vi "手动3界面.vi"(8 "错误输入（无错误）":errorcluster, 10 "界面切换队列":refnum<queue>, 11 "VISA资源名称输入":refnum<visa-resource-name>) -> (0 "错误输出":errorcluster, 3 "VISA资源名称输出":refnum<visa-resource-name>)   [LabVIEW 2018]
panel:
  out "DT470+上限+主料盘第三个":dbl
  out "DT469+下限+主料盘第三个":dbl
  out "DT468+上限+主料盘第二个":dbl
  out "DT467+下限+主料盘第二个":dbl
  out "R3":bool
  out "毫秒计时值":u32
  in  "枚举":T1(ring)
  in  "选项卡控件":enum32{"选项卡 1", "选项卡 2"}(tab)
  out "写R2E+读Y1C+2号吸嘴真空":bool
  out "写R2C+读Y1B+1号吸嘴真空":bool
  out "写R66+读R67+Z2下降取料":bool
  out "写R62+读R63+Z1下降取料":bool
  out "写R1F+读R5F+R2轴旋转定位":bool
  out "写R1C+读R5C+R1轴旋转定位":bool
  out "写R6C+读R6D+Z轴校正位取料":bool
  out "写R64+读R65+XYZ2到2号飞达位":bool
  out "写R60+读R61+XYZ1到飞达位":bool
  out "写R6A+读R6B+Z轴校正位放料":bool
  out "写R3F+读R4F+Z2下降编带":bool
  out "写R3D+读R4D+Z1下降编带":bool
  out "写R37+读R47+Z2下降取料":bool
  out "写R168+读R168+切换+快速":bool
  out "写R35+读R45+Z1下降取料":bool
  out "写R68+读R69+XY到校正位":bool
  out "写R3E+读R4E+XYZ2到2号编带位":bool
  out "写R3C+读R4C+XYZ1到1号编带位":bool
  out "写R36+读R46+XYZ2到指定点":bool
  out "写DT676+主料盘第3个":dbl
  out "写DT670+主料盘第2个":dbl
  out "写DDT600+主料盘已取个数":dbl
  out "手动2界面":bool
  out "DDT90356":dbl
  out "DDT90348":dbl
  out "自动界面":bool
  out "手动界面":bool
  out "参数界面":bool
  out "IO界面":bool
  out "产品界面":bool
  out "字符串":string
  out "DDT90352":dbl
  out "DDT90360":dbl
  out "DT1184":T2(ring)
  out "写R0+读R1+手动启动":bool
  out "写R4+读R4+手动停止":bool
  out "写R8+读R9+机器复位":bool
  out "写R80+读R80+报警清除":bool
  out "手动4界面":bool
  out "通讯周期":dbl
  in  "DT62+枚举":enum16{"90度", "180度", "270度"}(ring)
  in  "DT63+枚举":enum16{"90度", "180度", "270度"}(ring)
  out "写R76+读R76+主料盘修改":bool
  out "写R81+读R81+切换+快速":bool
  out "写R34+读R44+XYZ1到指定点":bool
  # "X"
  # "Z1"
  # "Z2"
  # "Y"
  # "备\n料\n盘\n状\n态"
  # "已取"
  # "个"
  # "第"
  # "行"
  # "第"
  # "个"
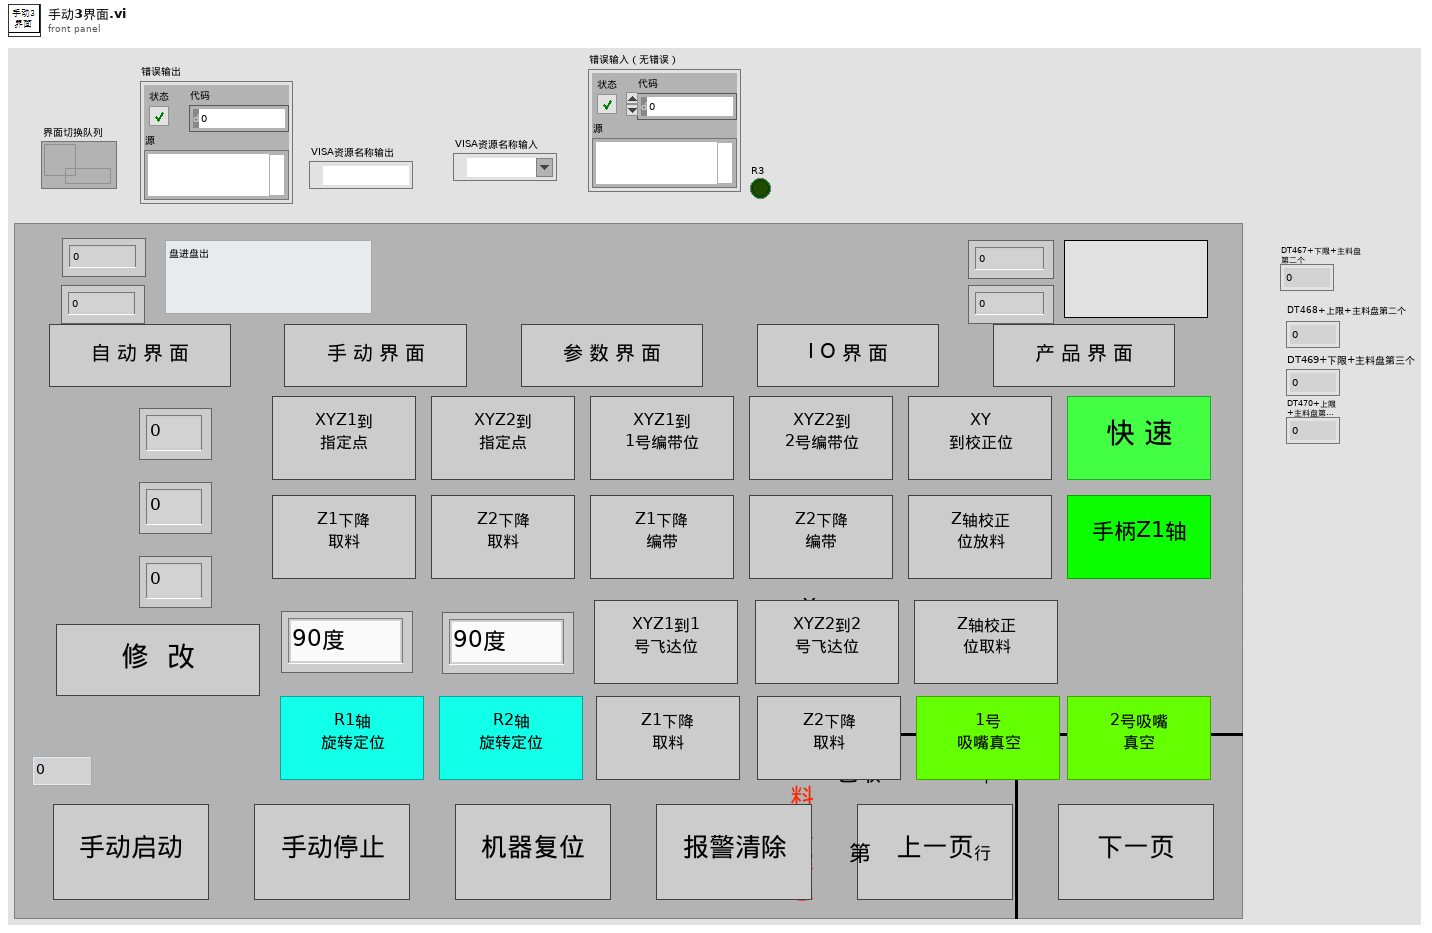
[diagram p1: front panel]
types:
  T1 = enum16{"读初始化", "读DT467+10", "读R4C+8", "读R44+8", "读R61+8", "读R75+8", "读R168+8", "读Y1B+8", "读R80+8", "读R69+8", "读R5C+8", "读R9+8", "读R1+8", "读DT670+10", "读DDT600+5", "读DT1184", "读DT62+10", "读DDT90356", "读DDT90348", ""}
  T2 = enum16{"盘进盘出", "卷进卷出", "盘进卷出", "管进盘出", "管进卷出", "卷进盘出", ""}
  T3 = typedef "数据簇.ctl" = cluster{"字符串":string, "数值":i32, "布尔":bool}
  T4 = enum8{"Enabled", "Disabled", "Disabled and Grayed Out"}
  T5 = typedef "lveventtype.ctl" = enum32{"Null", "Timeout", "Annotation Menu Selection", "Annotation Menu Selection?", "App Instance Close", "App Instance Close?", "Autoscale Range Change", "Bookmark Info Change", "Cell Edit", "Cell Edit?", "Cursor Grab", "Cursor Grab?", "Cursor Menu Selection", "Cursor Menu Selection?", "Cursor Move", "Cursor Release", "Data Change", "Direction Change", "Display State Change", "Drag Ended", "Drag Enter", "Drag Leave", "Drag Over", "Drag Source Update", "Drag Starting", "Drag Starting?", "Drop", "Exec State Change", "Key Down", "Key Down?", "Key Repeat", "Key Repeat?", "Key Up", "Listbox Double Click", "Menu Activation?", "Menu Selection (App)", "Menu Selection? (App)", "Menu Selection (User)", "Mouse Down", "Mouse Down?", "Mouse Enter", "Mouse Leave", "Mouse Move", "Mouse Up", "Mouse Wheel", "NI Security User Change (App)", "Pane Size", "Panel Close", "Panel Close?", "Panel Resize", "Plot Attribute Change", "Scale Range Change", "Shortcut Menu Activation?", "Shortcut Menu Selection (App)", "Shortcut Menu Selection? (App)", "Shortcut Menu Selection (User)", "Tree Double Click", "Tree Drag", "Tree Drag?", "Tree Drop", "Tree Drop?", "Tree Item Close", "Tree Item Close?", "Tree Item Open", "Tree Item Open?", "User Event", "Value Change"}
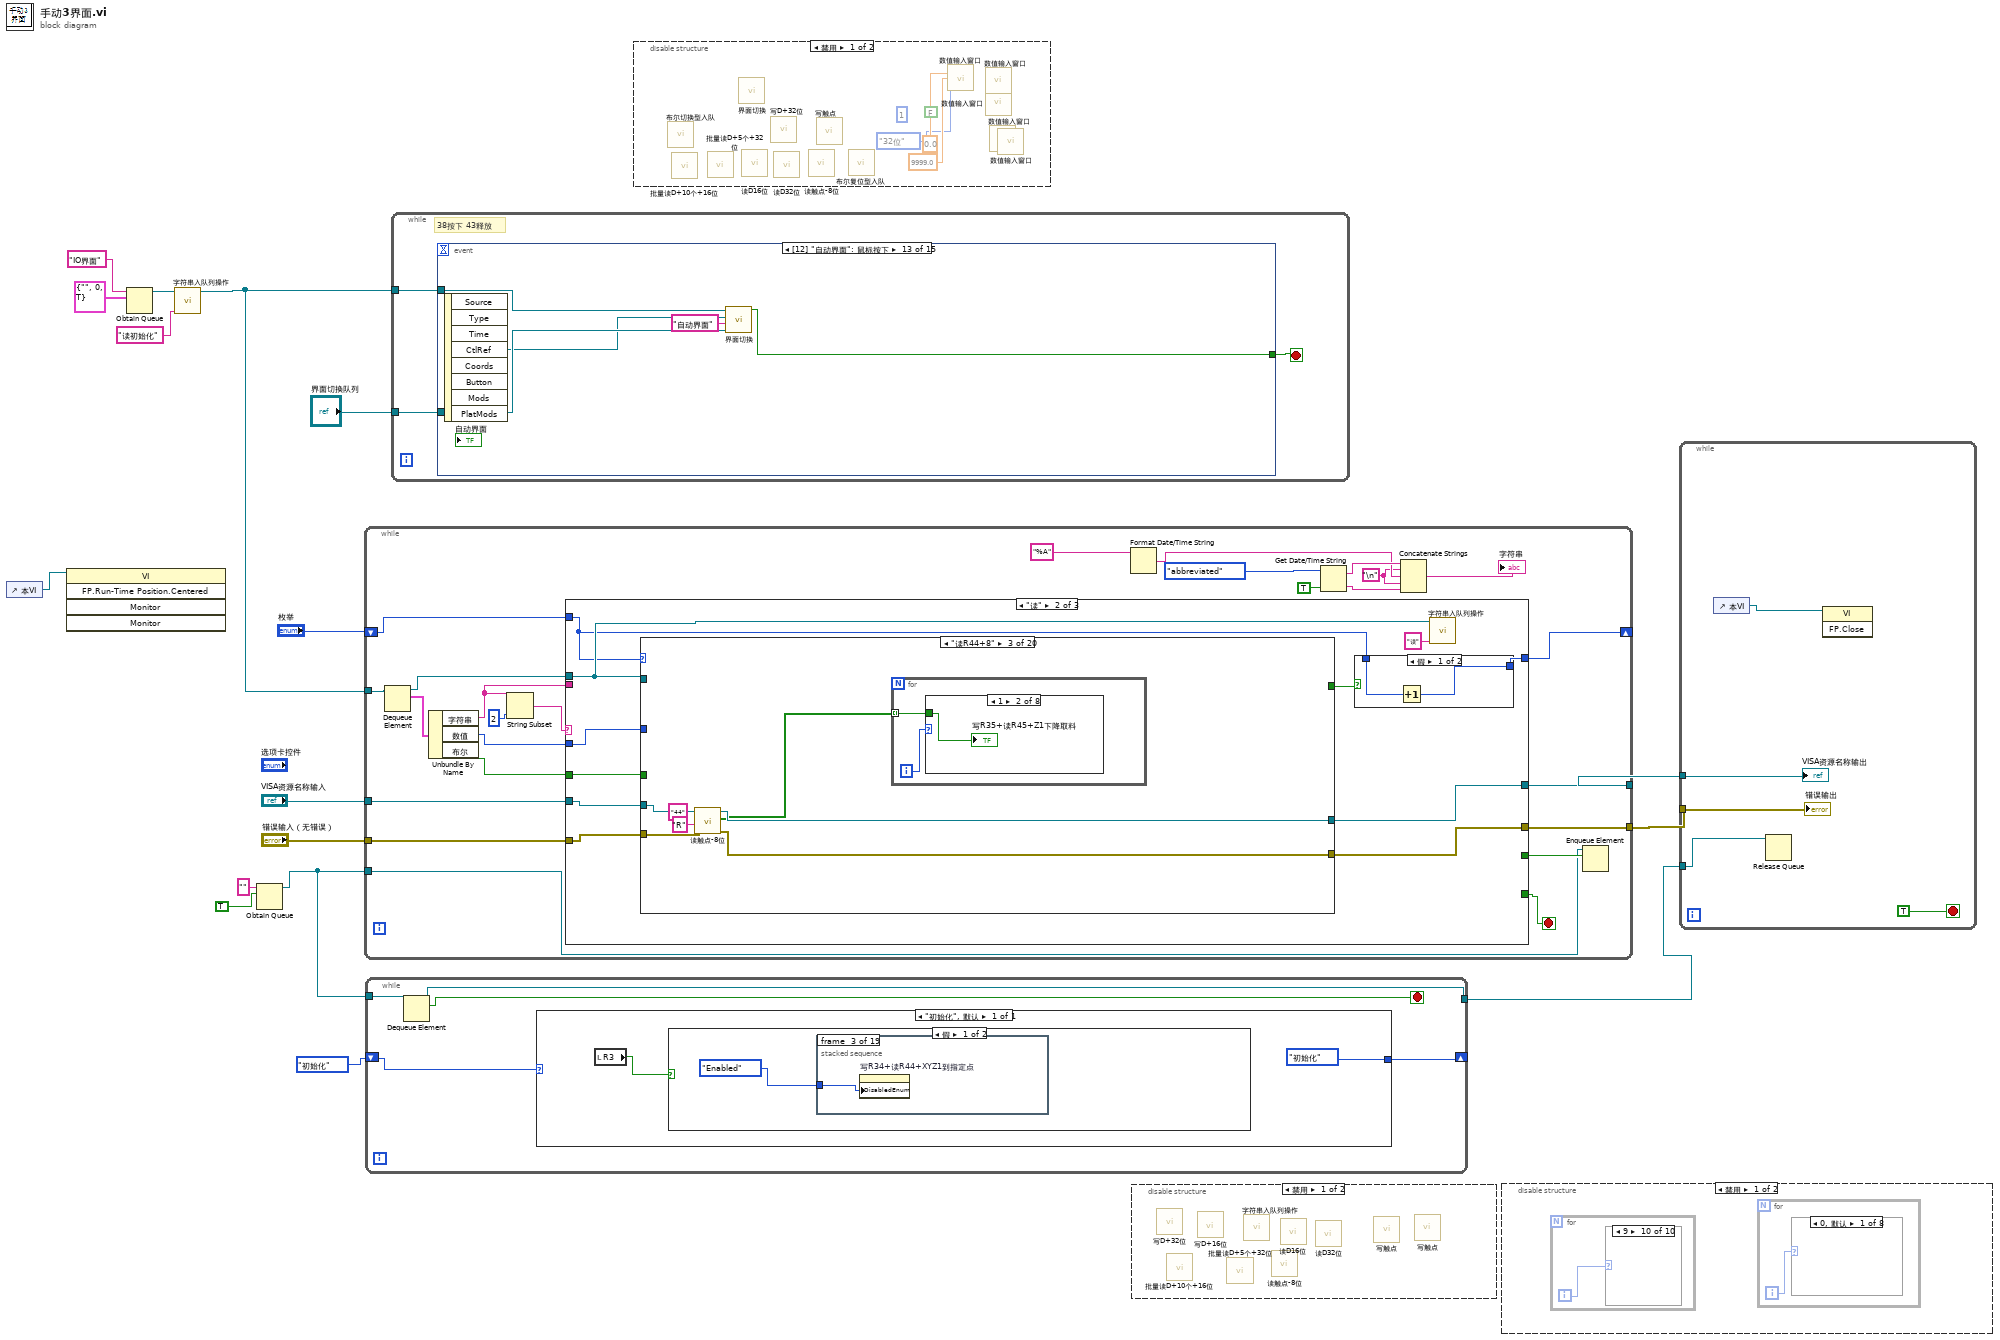
[diagram p0: block diagram]
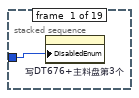
[diagram p2: hidden frame]
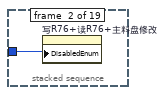
[diagram p3: hidden frame]
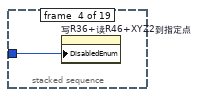
[diagram p4: hidden frame]
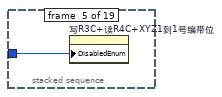
[diagram p5: hidden frame]
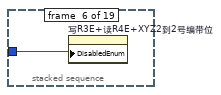
[diagram p6: hidden frame]
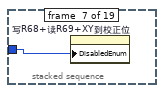
[diagram p7: hidden frame]
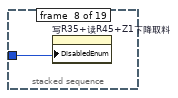
[diagram p8: hidden frame]
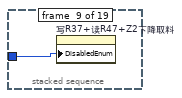
[diagram p9: hidden frame]
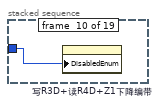
[diagram p10: hidden frame]
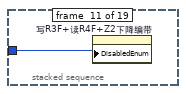
[diagram p11: hidden frame]
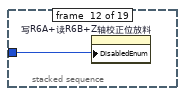
[diagram p12: hidden frame]
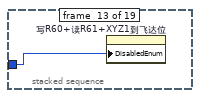
[diagram p13: hidden frame]
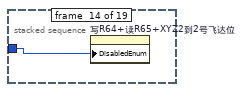
[diagram p14: hidden frame]
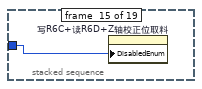
[diagram p15: hidden frame]
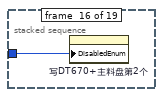
[diagram p16: hidden frame]
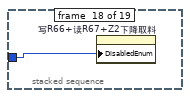
[diagram p18: hidden frame]
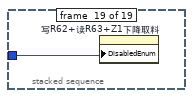
[diagram p19: hidden frame]
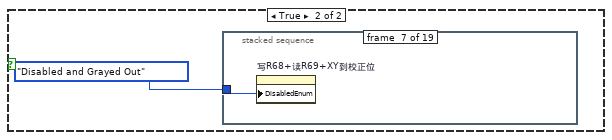
[diagram p20: hidden frame]
diagram:
  n1 = control-ref of="本VI"() -> (w2:refnum<vi>)
  n2 = invoke class="VI" method="FP.Run-Time Position.Centered"(reference=w2) -> ()  [unwired: 4 in, 5 out]
  n3 = Obtain Queue(name (unnamed)="IO界面" ("名称（未命名）"), element data type=T3 {"字符串"="", "数值"=0, "布尔"=TRUE}) -> (queue out=w10:refnum<queue>)  [unwired: 3 in, 2 out]
  n4 = call "字符串入队列操作.vi"("字符消息入队列"="读初始化", "界面切换队列"=w10) -> ("队列输出"=w3:refnum<queue>)  [unwired: 9 in]
  n5 = Obtain Queue(name (unnamed)="" ("名称（未命名）"), element data type=TRUE) -> (queue out=w6:refnum<queue>)  [unwired: 3 in, 2 out]
  n6 = while {
    tunnel: w3 -> [w38]
    tunnel: "VISA资源名称输入" -> [w31]
    tunnel: "错误输入（无错误）" -> [w30]
    tunnel: [w29] -> w12
    tunnel: [w28] -> w11
    shift-right: [w25] -> _
    shift-left: "枚举" -> [w26]
    tunnel: w6 -> [w18]
    stop <- w20 stop-if-true
    w22 = "\n"
    n7 = Dequeue Element(queue=w38) -> (queue out=w35:refnum<queue>, element=w37:T3)  [unwired: 2 in, 2 out]
    n8 = Unbundle By Name(w37) -> ("字符串"=w32:string, "数值"=w34:i32, "布尔"=w33:bool)
    n9 = String Subset(string=w32, length (rest)=2 ("长度（剩余）")) -> (substring=w36:string)  [unwired: 1 in]
    n10 = case shown="\"读\"" w36 {
      selector: w36 -> [w45 _ _]
      tunnel: w35 -> [_ w53 w290]
      tunnel: w34 -> [_ w60 w289]
      tunnel: w33 -> [_ w59 w288]
      tunnel: w32 -> [_ _ w282]
      tunnel: w31 -> [w44 w58 w287]
      tunnel: w30 -> [w43 w57 w286]
      tunnel: [w44 w56 w284] -> w29
      tunnel: [w43 w55 w283] -> w28
      tunnel: [_ _ w285] -> w20
      tunnel: w26 -> [_ w51 _]
      tunnel: [_ w50 _] -> w25
      tunnel: [_ _ w280] -> w19
      frame "", Default {
        n11 = Concatenate Strings("无对应消息分支**" ("消息"), w45, "**" ("字符串"), "读写状态机" ("字符串")) -> (w47:string)
        n12 = One Button Dialog(message=w47) -> ()  [unwired: 1 in, 1 out]
      }
      frame "读" {
        n13 = case shown="\"读R44+8\"" w51 {
          tunnel: w53 -> [_ _ _ _ _ _ _ _ _ _ _ _ _ _ _ _ _ _ _ _]
          tunnel: w60 -> [_ _ _ _ _ _ _ _ _ _ _ _ _ _ _ _ _ _ _ _]
          tunnel: w58 -> [w65 w72 w85 w98 w111 w121 w131 w142 w153 w165 w176 w186 w198 w208 w216 w223 w239 w255 w267 w273]
          tunnel: w57 -> [w64 w71 w84 w97 w110 w120 w130 w141 w152 w164 w175 w185 w197 w207 w215 w222 w238 w254 w266 w272]
          tunnel: [w65 w68 w81 w96 w109 w119 w127 w140 w151 w163 w174 w184 w195 w205 w214 w220 w237 w253 w267 w270] -> w56
          tunnel: [w64 w67 w80 w95 w108 w118 w126 w139 w150 w162 w173 w183 w194 w204 w213 w219 w236 w252 w266 w269] -> w55
          tunnel: w59 -> [_ _ _ _ _ _ _ _ _ _ _ _ _ _ _ _ _ _ _ _]
          tunnel: [_ _ _ _ _ _ _ _ _ _ _ _ _ _ _ _ _ _ TRUE _] -> w52
          frame "读初始化" {
            n14 = Tick Count (ms)() -> (millisecond timer value=→"毫秒计时值":u32)
          }
          frame "读R4C+8" {
            n15 = call "读触点-8位.vi"("error out"=w71, "触点类型"="R", "读取起始地址"="4C", "VISA resource name out"=w72) -> ("error IO"=w67:errorcluster, "读取布尔数组"=w66:bool[], "VISA resource name out 2"=w68:refnum<visa-resource-name>)  [unwired: 4 in, 1 out]
            n16 = for {
              tunnel: w66 -> [w73] mode=indexing
              i -> [w74]
              n17 = case shown="3" w74 {
                tunnel: w73 -> [w75 w76 w77 w78 _ _ _ _]
                frame 0, Default {
                  "写R3C+读R4C+XYZ1到1号编带位" <- w75
                }
                frame 1 {
                  "写R3D+读R4D+Z1下降编带" <- w76
                }
                frame 2 {
                  "写R3E+读R4E+XYZ2到2号编带位" <- w77
                }
                frame 3 {
                  "写R3F+读R4F+Z2下降编带" <- w78
                }
                frame 4 {
                }
                frame 5 {
                }
                frame 6 {
                }
                frame 7 {
                }
              }
            }
          }
          frame "读R44+8" {
            n18 = call "读触点-8位.vi"("error out"=w84, "触点类型"="R", "读取起始地址"="44", "VISA resource name out"=w85) -> ("error IO"=w80:errorcluster, "读取布尔数组"=w79:bool[], "VISA resource name out 2"=w81:refnum<visa-resource-name>)  [unwired: 4 in, 1 out]
            n19 = for {
              tunnel: w79 -> [w86] mode=indexing
              i -> [w87]
              n20 = case shown="1" w87 {
                tunnel: w86 -> [w88 w89 w90 w91 _ _ _ _]
                frame 0, Default {
                  "写R34+读R44+XYZ1到指定点" <- w88
                }
                frame 1 {
                  "写R35+读R45+Z1下降取料" <- w89
                }
                frame 2 {
                  "写R36+读R46+XYZ2到指定点" <- w90
                }
                frame 3 {
                  "写R37+读R47+Z2下降取料" <- w91
                }
                frame 4 {
                }
                frame 5 {
                }
                frame 6 {
                }
                frame 7 {
                }
              }
            }
          }
          frame "读R61+8" {
            n21 = call "读触点-8位.vi"("error out"=w97, "触点类型"="R", "读取起始地址"="61", "VISA resource name out"=w98) -> ("error IO"=w95:errorcluster, "读取布尔数组"=w92:bool[], "VISA resource name out 2"=w96:refnum<visa-resource-name>)  [unwired: 4 in, 1 out]
            n22 = for {
              tunnel: w92 -> [w99] mode=indexing
              i -> [w100]
              n23 = case shown="6" w100 {
                tunnel: w99 -> [w101 _ w102 _ w103 _ w104 _]
                frame 0, Default {
                  "写R60+读R61+XYZ1到飞达位" <- w101
                }
                frame 1 {
                }
                frame 2 {
                  "写R62+读R63+Z1下降取料" <- w102
                }
                frame 3 {
                }
                frame 4 {
                  "写R64+读R65+XYZ2到2号飞达位" <- w103
                }
                frame 5 {
                }
                frame 6 {
                  "写R66+读R67+Z2下降取料" <- w104
                }
                frame 7 {
                }
              }
            }
          }
          frame "读R75+8" {
            n24 = call "读触点-8位.vi"("error out"=w110, "触点类型"="R", "读取起始地址"="75", "VISA resource name out"=w111) -> ("error IO"=w108:errorcluster, "读取布尔数组"=w105:bool[], "VISA resource name out 2"=w109:refnum<visa-resource-name>)  [unwired: 4 in, 1 out]
            n25 = for {
              tunnel: w105 -> [w112] mode=indexing
              i -> [w113]
              n26 = case shown="0, 默认" w113 {
                tunnel: w112 -> [w114 _ _ _ _ _ _ _]
                frame 0, Default {
                  "写R76+读R76+主料盘修改" <- w114
                }
                frame 1 {
                }
                frame 2 {
                }
                frame 3 {
                }
                frame 4 {
                }
                frame 5 {
                }
                frame 6 {
                }
                frame 7 {
                }
              }
            }
          }
          frame "读R168+8" {
            n27 = call "读触点-8位.vi"("error out"=w120, "触点类型"="R", "读取起始地址"="168", "VISA resource name out"=w121) -> ("error IO"=w118:errorcluster, "读取布尔数组"=w115:bool[], "VISA resource name out 2"=w119:refnum<visa-resource-name>)  [unwired: 4 in, 1 out]
            n28 = for {
              tunnel: w115 -> [w122] mode=indexing
              i -> [w123]
              n29 = case shown="0, 默认" w123 {
                tunnel: w122 -> [w124 _ _ _ _ _ _ _]
                frame 0, Default {
                  "写R168+读R168+切换+快速" <- w124
                }
                frame 1 {
                }
                frame 2 {
                }
                frame 3 {
                }
                frame 4 {
                }
                frame 5 {
                }
                frame 6 {
                }
                frame 7 {
                }
              }
            }
          }
          frame "读Y1B+8" {
            n30 = call "读触点-8位.vi"("error out"=w130, "触点类型"="Y", "读取起始地址"="1B", "VISA resource name out"=w131) -> ("error IO"=w126:errorcluster, "读取布尔数组"=w125:bool[], "VISA resource name out 2"=w127:refnum<visa-resource-name>)  [unwired: 4 in, 1 out]
            n31 = for {
              tunnel: w125 -> [w132] mode=indexing
              i -> [w133]
              n32 = case shown="1" w133 {
                tunnel: w132 -> [w134 w135 _ _ _ _ _ _]
                frame 0, Default {
                  "写R2C+读Y1B+1号吸嘴真空" <- w134
                }
                frame 1 {
                  "写R2E+读Y1C+2号吸嘴真空" <- w135
                }
                frame 2 {
                }
                frame 3 {
                }
                frame 4 {
                }
                frame 5 {
                }
                frame 6 {
                }
                frame 7 {
                }
              }
            }
          }
          frame "读R80+8" {
            n33 = call "读触点-8位.vi"("error out"=w141, "触点类型"="R", "读取起始地址"="80", "VISA resource name out"=w142) -> ("error IO"=w139:errorcluster, "读取布尔数组"=w136:bool[], "VISA resource name out 2"=w140:refnum<visa-resource-name>)  [unwired: 4 in, 1 out]
            n34 = for {
              tunnel: w136 -> [w143] mode=indexing
              i -> [w144]
              n35 = case shown="1" w144 {
                tunnel: w143 -> [w145 w146 _ _ _ _ _ _]
                frame 0, Default {
                  "写R80+读R80+报警清除" <- w145
                }
                frame 1 {
                  "写R81+读R81+切换+快速" <- w146
                }
                frame 2 {
                }
                frame 3 {
                }
                frame 4 {
                }
                frame 5 {
                }
                frame 6 {
                }
                frame 7 {
                }
              }
            }
          }
          frame "读R69+8" {
            n36 = call "读触点-8位.vi"("error out"=w152, "触点类型"="R", "读取起始地址"="69", "VISA resource name out"=w153) -> ("error IO"=w150:errorcluster, "读取布尔数组"=w149:bool[], "VISA resource name out 2"=w151:refnum<visa-resource-name>)  [unwired: 4 in, 1 out]
            n37 = for {
              tunnel: w149 -> [w154] mode=indexing
              i -> [w155]
              n38 = case shown="4" w155 {
                tunnel: w154 -> [w156 _ w157 _ w158 _ _ _]
                frame 0, Default {
                  "写R68+读R69+XY到校正位" <- w156
                }
                frame 1 {
                }
                frame 2 {
                  "写R6A+读R6B+Z轴校正位放料" <- w157
                }
                frame 3 {
                }
                frame 4 {
                  "写R6C+读R6D+Z轴校正位取料" <- w158
                }
                frame 5 {
                }
                frame 6 {
                }
                frame 7 {
                }
              }
            }
          }
          frame "读R5C+8" {
            n39 = call "读触点-8位.vi"("error out"=w164, "触点类型"="R", "读取起始地址"="5C", "VISA resource name out"=w165) -> ("error IO"=w162:errorcluster, "读取布尔数组"=w161:bool[], "VISA resource name out 2"=w163:refnum<visa-resource-name>)  [unwired: 4 in, 1 out]
            n40 = for {
              tunnel: w161 -> [w166] mode=indexing
              i -> [w167]
              n41 = case shown="3" w167 {
                tunnel: w166 -> [w168 _ _ w169 _ _ _ _]
                frame 0, Default {
                  "写R1C+读R5C+R1轴旋转定位" <- w168
                }
                frame 1 {
                }
                frame 2 {
                }
                frame 3 {
                  "写R1F+读R5F+R2轴旋转定位" <- w169
                }
                frame 4 {
                }
                frame 5 {
                }
                frame 6 {
                }
                frame 7 {
                }
              }
            }
          }
          frame "读R9+8" {
            n42 = call "读触点-8位.vi"("error out"=w175, "触点类型"="R", "读取起始地址"="9", "VISA resource name out"=w176) -> ("error IO"=w173:errorcluster, "读取布尔数组"=w170:bool[], "VISA resource name out 2"=w174:refnum<visa-resource-name>)  [unwired: 4 in, 1 out]
            n43 = for {
              tunnel: w170 -> [w177] mode=indexing
              i -> [w178]
              n44 = case shown="0, 默认" w178 {
                tunnel: w177 -> [w179 _ _ _ _ _ _ _]
                frame 0, Default {
                  "写R8+读R9+机器复位" <- w179
                }
                frame 1 {
                }
                frame 2 {
                }
                frame 3 {
                }
                frame 4 {
                }
                frame 5 {
                }
                frame 6 {
                }
                frame 7 {
                }
              }
            }
          }
          frame "读R1+8" {
            n45 = call "读触点-8位.vi"("error out"=w185, "触点类型"="R", "读取起始地址"="1", "VISA resource name out"=w186) -> ("error IO"=w183:errorcluster, "读取布尔数组"=w180:bool[], "VISA resource name out 2"=w184:refnum<visa-resource-name>)  [unwired: 4 in, 1 out]
            n46 = for {
              tunnel: w180 -> [w187] mode=indexing
              i -> [w188]
              n47 = case shown="2" w188 {
                tunnel: w187 -> [w189 _ w190 w192 _ _ _ _]
                frame 0, Default {
                  "写R0+读R1+手动启动" <- w189
                }
                frame 1 {
                }
                frame 2 {
                  # "R3"
                  n48 = case shown="假" w190 {
                    selector: w190 -> [w191 _]
                    frame False {
                      "R3" <- w191
                    }
                    frame True {
                      (unwired) T4."Disabled and Grayed Out" ("禁用")
                    }
                  }
                }
                frame 3 {
                  "写R4+读R4+手动停止" <- w192
                }
                frame 4 {
                }
                frame 5 {
                }
                frame 6 {
                }
                frame 7 {
                }
              }
            }
          }
          frame "读DT670+10" {
            n49 = call "批量读D+10个+16位.vi"("error out"=w197, "读取D地址"=670, "VISA resource name out"=w198) -> ("error IO"=w194:errorcluster, "数组"=w193:i32[], "VISA resource name out 2"=w195:refnum<visa-resource-name>)  [unwired: 5 in, 1 out]
            n50 = for {
              tunnel: w193 -> [w199] mode=indexing
              i -> [w200]
              n51 = case shown="0, 默认" w200 {
                tunnel: w199 -> [w201 _ _ _ _ _ w202 _ _ _]
                frame 0, Default {
                  "写DT670+主料盘第2个" <- w201
                }
                frame 1 {
                }
                frame 2 {
                }
                frame 3 {
                }
                frame 4 {
                }
                frame 5 {
                }
                frame 6 {
                  "写DT676+主料盘第3个" <- w202
                }
                frame 7 {
                }
                frame 8 {
                }
                frame 9 {
                }
              }
            }
          }
          frame "读DDT600+5" {
            n52 = call "批量读D+5个+32位.vi"("error out"=w207, "读取D地址"=600, "VISA resource name out"=w208) -> ("error IO"=w204:errorcluster, "数组"=w203:i32[], "VISA resource name out 2"=w205:refnum<visa-resource-name>)  [unwired: 5 in, 1 out]
            n53 = for {
              tunnel: w203 -> [w209] mode=indexing
              i -> [w210]
              n54 = case shown="4" w210 {
                tunnel: w209 -> [w211 _ _ _ _]
                frame 0, Default {
                  "写DDT600+主料盘已取个数" <- w211
                }
                frame 1 {
                }
                frame 2 {
                }
                frame 3 {
                }
                frame 4 {
                }
              }
            }
          }
          frame "读DT1184" {
            n55 = call "读D16位.vi"("error out"=w215, "读取D地址"=1184, "VISA resource name out"=w216) -> ("error IO"=w213:errorcluster, "数值"=→"DT1184":u32, "VISA resource name out 2"=w214:refnum<visa-resource-name>)  [unwired: 5 in, 1 out]
          }
          frame "读DT62+10" {
            n56 = call "批量读D+10个+16位.vi"("error out"=w222, "读取D地址"=62, "VISA resource name out"=w223) -> ("error IO"=w219:errorcluster, "数组"=w218:i32[], "VISA resource name out 2"=w220:refnum<visa-resource-name>)  [unwired: 5 in, 1 out]
            n57 = for {
              tunnel: w218 -> [w224] mode=indexing
              i -> [w225]
              n58 = case shown="1" w225 {
                tunnel: w224 -> [w226 w227 _ _ _ _ _ _]
                frame 0, Default {
                  n59 = local write "DT62+枚举"(w226) -> ()
                }
                frame 1 {
                  n60 = local write "DT63+枚举"(w227) -> ()
                }
                frame 2 {
                }
                frame 3 {
                }
                frame 4 {
                }
                frame 5 {
                }
                frame 6 {
                }
                frame 7 {
                }
              }
            }
          }
          frame "读DDT90356" {
            n61 = call "批量读D+5个+32位.vi"("error out"=w238, "读取D地址"=90356, "VISA resource name out"=w239) -> ("error IO"=w236:errorcluster, "数组"=w242:i32[], "VISA resource name out 2"=w237:refnum<visa-resource-name>)  [unwired: 5 in, 1 out]
            n62 = Index Array(array=w242, index #1=0 ("索引"), index #2=2 ("索引")) -> (element #1=w235:i32, element #2=w234:i32)
            n63 = To Double Precision Float(number=w235) -> (double precision float=w233:dbl)
            n64 = To Double Precision Float(number=w234) -> (double precision float=w230:dbl)
            n65 = Divide(x=w233, y=100.0) -> (x/y=→"DDT90356":dbl)
            n66 = Divide(x=w230, y=100.0) -> (x/y=→"DDT90360":dbl)
          }
          frame "读DDT90348" {
            n67 = call "批量读D+5个+32位.vi"("error out"=w254, "读取D地址"=90348, "VISA resource name out"=w255) -> ("error IO"=w252:errorcluster, "数组"=w259:i32[], "VISA resource name out 2"=w253:refnum<visa-resource-name>)  [unwired: 5 in, 1 out]
            n68 = Index Array(array=w259, index #1=0 ("索引"), index #2=2 ("索引")) -> (element #1=w251:i32, element #2=w250:i32)
            n69 = To Double Precision Float(number=w250) -> (double precision float=w245:dbl)
            n70 = To Double Precision Float(number=w251) -> (double precision float=w249:dbl)
            n71 = Divide(x=w245, y=100.0) -> (x/y=→"DDT90352":dbl)
            n72 = Divide(x=w249, y=100.0) -> (x/y=→"DDT90348":dbl)
          }
          frame "" {
            n73 = local read "毫秒计时值"() -> (w263:u32)
            n74 = Tick Count (ms)() -> (millisecond timer value=w264:u32)
            n75 = Subtract(x=w264, y=w263) -> (x-y=w262:u32)
            n76 = Divide(x=w262, y=u32 1000) -> (x/y=→"通讯周期":dbl)
          }
          frame "读DT467+10" {
            n77 = call "批量读D+10个+16位.vi"("error out"=w272, "读取D地址"=467, "VISA resource name out"=w273) -> ("error IO"=w269:errorcluster, "数组"=w268:i32[], "VISA resource name out 2"=w270:refnum<visa-resource-name>)  [unwired: 5 in, 1 out]
            n78 = for {
              tunnel: w268 -> [w274] mode=indexing
              i -> [w275]
              n79 = case shown="3" w275 {
                tunnel: w274 -> [w276 w277 w278 w279 _ _ _ _]
                frame 0, Default {
                  "DT467+下限+主料盘第二个" <- w276
                }
                frame 1 {
                  "DT468+上限+主料盘第二个" <- w277
                }
                frame 2 {
                  "DT469+下限+主料盘第三个" <- w278
                }
                frame 3 {
                  "DT470+上限+主料盘第三个" <- w279
                }
                frame 4 {
                }
                frame 5 {
                }
                frame 6 {
                }
                frame 7 {
                }
              }
            }
          }
        }
        n80 = case shown="假" w52 {
          tunnel: w51 -> [w62 _]
          tunnel: [w61 _] -> w50
          frame False {
            n81 = Increment(x=w62) -> (x+1=w61:T1)
          }
          frame True {
          }
        }
        n82 = call "字符串入队列操作.vi"("字符消息入队列"="读", "界面切换队列"=w53) -> ()  [unwired: 9 in, 1 out]
      }
      frame "写" {
        n83 = call "状态匹配.vi"("输入状态"=w282) -> ("输出状态"=w281:string)  [unwired: 10 in]
        n84 = case shown="\"写退出\"" w281 {
          selector: w281 -> [w293 _ _ _ _]
          tunnel: w290 -> [_ _ _ _ w333]
          tunnel: w289 -> [_ w299 w316 _ _]
          tunnel: w288 -> [_ _ _ w327 _]
          tunnel: w287 -> [w292 w309 w320 w332 w338]
          tunnel: w286 -> [w291 w308 w319 w331 w337]
          tunnel: [_ _ _ _ w336] -> w285
          tunnel: [w292 w307 w318 w330 w338] -> w284
          tunnel: [w291 w306 w317 w329 w337] -> w283
          tunnel: w282 -> [_ w298 w310 w321 _]
          tunnel: [_ _ _ _ w336] -> w280
          frame "", Default {
            n85 = Concatenate Strings("无对应消息分支**" ("消息"), w293, "**" ("字符串"), "写状态机" ("字符串")) -> (w297:string)
            n86 = One Button Dialog(message=w297) -> ()  [unwired: 1 in, 1 out]
          }
          frame "写DT" {
            n87 = String Length(string=w298) -> (length=w304:i32)
            n88 = Subtract(x=w304, y=4) -> (x-y=w302:i32)
            n89 = String Subset(string=w298, offset (0)=4 ("偏移量(0)"), length (rest)=w302) -> (substring=w301:string)
            n90 = Decimal String To Number(string=w301) -> (number=w300:i32)  [unwired: 2 in, 1 out]
            n91 = call "写D+16位.vi"("error out"=w308, "输入数值"=w299, "输入地址D"=w300, "VISA resource name out"=w309) -> ("error out 2"=w306:errorcluster, "VISA resource name out 2"=w307:refnum<visa-resource-name>)  [unwired: 3 in, 3 out]
          }
          frame "写DDT" {
            n92 = String Length(string=w310) -> (length=w314:i32)
            n93 = Subtract(x=w314, y=5) -> ()  [unwired: 1 out]
            n94 = String Subset(string=w310, offset (0)=5 ("偏移量(0)")) -> (substring=w311:string)  [unwired: 1 in]
            n95 = Decimal String To Number(string=w311) -> (number=w312:i32)  [unwired: 2 in, 1 out]
            n96 = call "写D+32位.vi"("error out"=w319, "输入数值"=w316, "输入地址D"=w312, "VISA resource name out"=w320) -> ("error out 2"=w317:errorcluster, "VISA resource name out 2"=w318:refnum<visa-resource-name>)  [unwired: 4 in, 2 out]
          }
          frame "写R" {
            n97 = String Length(string=w321) -> (length=w325:i32)
            n98 = Subtract(x=w325, y=3) -> (x-y=w323:i32)
            n99 = String Subset(string=w321, offset (0)=3 ("偏移量(0)"), length (rest)=w323) -> (substring=w322:string)
            n100 = call "写触点.vi"("布尔"=w327, "error out"=w331, "触点类型"="R", "写入起始地址"=w322, "VISA resource name out"=w332) -> ("error IO"=w329:errorcluster, "VISA resource name out 2"=w330:refnum<visa-resource-name>)  [unwired: 4 in, 1 out]
          }
          frame "写退出" {
            w336 = TRUE
            n101 = Flush Queue(queue=w333) -> (queue out=w334:refnum<queue>, error out=w335:errorcluster)  [unwired: 1 in, 1 out]
            n102 = Release Queue(queue=w334, error in (no error)=w335) -> ()  [unwired: 1 in, 3 out]
          }
        }
      }
    }
    n103 = Format Date/Time String(time format string (%c)="%A" ("时间格式字符串(%c)")) -> (date/time string=w23:string)  [unwired: 2 in]
    n104 = Get Date/Time String(date format (0)=enum16{"short", "long", "abbreviated"}."abbreviated" ("日期格式(0)"), want seconds? (F)=TRUE ("需要秒？(F)")) -> (date string=w40:string, time string=w21:string)  [unwired: 1 in]
    n105 = Concatenate Strings(w40, w22, w23, w22, w21) -> (→"字符串":string)
    n106 = Enqueue Element(queue=w18, element=w19) -> ()  [unwired: 2 in, 3 out]
  }
  n107 = while {
    shift-right: [w342] -> _
    shift-left: enum16{"初始化"}."初始化" -> [w343]
    tunnel: w6 -> [w341]
    tunnel: [w339] -> w5
    stop <- w340 stop-if-true
    n108 = Dequeue Element(queue=w341) -> (queue out=w339:refnum<queue>, element=w340:bool)  [unwired: 2 in, 2 out]
    n109 = case shown="\"初始化\", 默认" w343 {
      tunnel: [enum16{"初始化"}."初始化"] -> w342
      frame "初始化", Default {
        n110 = local read "R3"() -> (w344:bool)
        n111 = case shown="假" w344 {
          frame False {
            n112 = stacked-sequence {
              tunnel: T4."Enabled" ("禁用") -> [w347 w348 w349 w350 w351 w352 w353 w354 w355 w356 w357 w358 w359 w360 w361 w362 _ w363 w364]
              frame #0 {
                n113 = property on="写DT676+主料盘第3个" class="DigNum (严格)"("DisabledEnum"=w347) -> ()  [unwired: 2 in, 2 out]
              }
              frame #1 {
                n114 = property on="写R76+读R76+主料盘修改" class="Bool"("DisabledEnum"=w348) -> ()  [unwired: 2 in, 2 out]
              }
              frame #2 {
                n115 = property on="写R34+读R44+XYZ1到指定点" class="Bool"("DisabledEnum"=w349) -> ()  [unwired: 2 in, 2 out]
              }
              frame #3 {
                n116 = property on="写R36+读R46+XYZ2到指定点" class="Bool"("DisabledEnum"=w350) -> ()  [unwired: 2 in, 2 out]
              }
              frame #4 {
                n117 = property on="写R3C+读R4C+XYZ1到1号编带位" class="Bool"("DisabledEnum"=w351) -> ()  [unwired: 2 in, 2 out]
              }
              frame #5 {
                n118 = property on="写R3E+读R4E+XYZ2到2号编带位" class="Bool"("DisabledEnum"=w352) -> ()  [unwired: 2 in, 2 out]
              }
              frame #6 {
                n119 = property on="写R68+读R69+XY到校正位" class="Bool"("DisabledEnum"=w353) -> ()  [unwired: 2 in, 2 out]
              }
              frame #7 {
                n120 = property on="写R35+读R45+Z1下降取料" class="Bool"("DisabledEnum"=w354) -> ()  [unwired: 2 in, 2 out]
              }
              frame #8 {
                n121 = property on="写R37+读R47+Z2下降取料" class="Bool"("DisabledEnum"=w355) -> ()  [unwired: 2 in, 2 out]
              }
              frame #9 {
                n122 = property on="写R3D+读R4D+Z1下降编带" class="Bool"("DisabledEnum"=w356) -> ()  [unwired: 2 in, 2 out]
              }
              frame #10 {
                n123 = property on="写R3F+读R4F+Z2下降编带" class="Bool"("DisabledEnum"=w357) -> ()  [unwired: 2 in, 2 out]
              }
              frame #11 {
                n124 = property on="写R6A+读R6B+Z轴校正位放料" class="Bool"("DisabledEnum"=w358) -> ()  [unwired: 2 in, 2 out]
              }
              frame #12 {
                n125 = property on="写R60+读R61+XYZ1到飞达位" class="Bool"("DisabledEnum"=w359) -> ()  [unwired: 2 in, 2 out]
              }
              frame #13 {
                n126 = property on="写R64+读R65+XYZ2到2号飞达位" class="Bool"("DisabledEnum"=w360) -> ()  [unwired: 2 in, 2 out]
              }
              frame #14 {
                n127 = property on="写R6C+读R6D+Z轴校正位取料" class="Bool"("DisabledEnum"=w361) -> ()  [unwired: 2 in, 2 out]
              }
              frame #15 {
                n128 = property on="写DT670+主料盘第2个" class="DigNum (严格)"("DisabledEnum"=w362) -> ()  [unwired: 2 in, 2 out]
              }
              frame #16 {
              }
              frame #17 {
                n129 = property on="写R66+读R67+Z2下降取料" class="Bool"("DisabledEnum"=w363) -> ()  [unwired: 2 in, 2 out]
              }
              frame #18 {
                n130 = property on="写R62+读R63+Z1下降取料" class="Bool"("DisabledEnum"=w364) -> ()  [unwired: 2 in, 2 out]
              }
            }
          }
          frame True {
            n131 = stacked-sequence {
              tunnel: T4."Disabled and Grayed Out" ("禁用") -> [w366 w367 w368 w369 w370 w371 w372 w373 w374 w375 w376 w377 w378 w379 w380 w381 _ w382 w383]
              frame #0 {
                n132 = property on="写DT676+主料盘第3个" class="DigNum (严格)"("DisabledEnum"=w366) -> ()  [unwired: 2 in, 2 out]
              }
              frame #1 {
                n133 = property on="写R76+读R76+主料盘修改" class="Bool"("DisabledEnum"=w367) -> ()  [unwired: 2 in, 2 out]
              }
              frame #2 {
                n134 = property on="写R34+读R44+XYZ1到指定点" class="Bool"("DisabledEnum"=w368) -> ()  [unwired: 2 in, 2 out]
              }
              frame #3 {
                n135 = property on="写R36+读R46+XYZ2到指定点" class="Bool"("DisabledEnum"=w369) -> ()  [unwired: 2 in, 2 out]
              }
              frame #4 {
                n136 = property on="写R3C+读R4C+XYZ1到1号编带位" class="Bool"("DisabledEnum"=w370) -> ()  [unwired: 2 in, 2 out]
              }
              frame #5 {
                n137 = property on="写R3E+读R4E+XYZ2到2号编带位" class="Bool"("DisabledEnum"=w371) -> ()  [unwired: 2 in, 2 out]
              }
              frame #6 {
                n138 = property on="写R68+读R69+XY到校正位" class="Bool"("DisabledEnum"=w372) -> ()  [unwired: 2 in, 2 out]
              }
              frame #7 {
                n139 = property on="写R35+读R45+Z1下降取料" class="Bool"("DisabledEnum"=w373) -> ()  [unwired: 2 in, 2 out]
              }
              frame #8 {
                n140 = property on="写R37+读R47+Z2下降取料" class="Bool"("DisabledEnum"=w374) -> ()  [unwired: 2 in, 2 out]
              }
              frame #9 {
                n141 = property on="写R3D+读R4D+Z1下降编带" class="Bool"("DisabledEnum"=w375) -> ()  [unwired: 2 in, 2 out]
              }
              frame #10 {
                n142 = property on="写R3F+读R4F+Z2下降编带" class="Bool"("DisabledEnum"=w376) -> ()  [unwired: 2 in, 2 out]
              }
              frame #11 {
                n143 = property on="写R6A+读R6B+Z轴校正位放料" class="Bool"("DisabledEnum"=w377) -> ()  [unwired: 2 in, 2 out]
              }
              frame #12 {
                n144 = property on="写R60+读R61+XYZ1到飞达位" class="Bool"("DisabledEnum"=w378) -> ()  [unwired: 2 in, 2 out]
              }
              frame #13 {
                n145 = property on="写R64+读R65+XYZ2到2号飞达位" class="Bool"("DisabledEnum"=w379) -> ()  [unwired: 2 in, 2 out]
              }
              frame #14 {
                n146 = property on="写R6C+读R6D+Z轴校正位取料" class="Bool"("DisabledEnum"=w380) -> ()  [unwired: 2 in, 2 out]
              }
              frame #15 {
                n147 = property on="写DT670+主料盘第2个" class="DigNum (严格)"("DisabledEnum"=w381) -> ()  [unwired: 2 in, 2 out]
              }
              frame #16 {
              }
              frame #17 {
                n148 = property on="写R66+读R67+Z2下降取料" class="Bool"("DisabledEnum"=w382) -> ()  [unwired: 2 in, 2 out]
              }
              frame #18 {
                n149 = property on="写R62+读R63+Z1下降取料" class="Bool"("DisabledEnum"=w383) -> ()  [unwired: 2 in, 2 out]
              }
            }
          }
        }
      }
    }
  }
  n150 = while {
    tunnel: w3 -> [w385]
    tunnel: "界面切换队列" -> [w384]
    stop <- w386 stop-if-true
    # "38按下 43释放"
    n151 = event shown="[12] \"自动界面\": 鼠标按下" {
      selector: _ -> [_ _ _ _ _ _ _ _ _ _ _ _ _ _ _]
      dyn-events: _ -> [_ _ _ _ _ _ _ _ _ _ _ _ _ _ _]
      timeout: _ -> [_ _ _ _ _ _ _ _ _ _ _ _ _ _ _]
      tunnel: [w387 w394 _ _ _ _ _ _ w433 w438 w443 w448 w453 _ w460] -> w386
      tunnel: w385 -> [w391 w396 w399 w407 w410 w419 w429 w432 w437 w442 w447 w452 w457 _ w459]
      tunnel: w384 -> [w390 w395 _ _ _ _ _ _ w436 w441 w446 w451 w456 _ w458]
      event "IO界面": Mouse Down {
        n152 = event-data() -> ("CtlRef"=w389:refnum<vi>)  [unwired: 1 in, 7 out]
        n153 = call "界面切换.vi"("界面切换队列输入"=w390, "切换界面名称输入"="IO界面", "Bool引用句柄"=w389, "状态转移输入"=w391) -> ("布尔"=w387:bool)  [unwired: 7 in]
      }
      event "参数界面": Mouse Down {
        n154 = event-data() -> ("CtlRef"=w393:refnum<vi>)  [unwired: 1 in, 7 out]
        n155 = call "界面切换.vi"("界面切换队列输入"=w395, "切换界面名称输入"="参数界面", "Bool引用句柄"=w393, "状态转移输入"=w396) -> ("布尔"=w394:bool)  [unwired: 7 in]
      }
      event "DT62+枚举": Value Change {
        n156 = event-data() -> ("NewVal"=w398:enum16{"90度", "180度", "270度"})  [unwired: 1 in, 5 out]
        n157 = call "字符串入队列操作.vi"("字符消息入队列"="写DT62", "数值"=w398, "界面切换队列"=w399) -> ()  [unwired: 8 in, 1 out]
      }
      event "写DT676+主料盘第3个": Mouse Down {
        n158 = event-data() -> ("CtlRef"=w404:refnum<vi>)  [unwired: 1 in, 7 out]
        n159 = local read "DT470+上限+主料盘第三个"() -> (w400:dbl)
        n160 = local read "DT469+下限+主料盘第三个"() -> (w401:dbl)
        n161 = call "数值输入窗口.vi"("消息入队"=w407, "字符串"="备料盘第3个", "字符消息入队列"="写DT676", "输入下限"=w401, "输入上限"=w400, "转换比例"=u32 1, "数据类型"=enum16{"32位", "16位"}."16位", "控件引用"=w404) -> ()  [unwired: 5 in, 3 out]
      }
      event "写DT670+主料盘第2个": Mouse Down {
        n162 = event-data() -> ("CtlRef"=w411:refnum<vi>)  [unwired: 1 in, 7 out]
        n163 = local read "DT467+下限+主料盘第二个"() -> (w408:dbl)
        n164 = local read "DT468+上限+主料盘第二个"() -> (w409:dbl)
        n165 = call "数值输入窗口.vi"("消息入队"=w410, "字符串"="备料盘第2个", "字符消息入队列"="写DT670", "输入下限"=w408, "输入上限"=w409, "转换比例"=u32 1, "数据类型"=enum16{"32位", "16位"}."16位", "控件引用"=w411) -> ()  [unwired: 5 in, 3 out]
      }
      event "写R0+读R1+手动启动", "写R4+读R4+手动停止", "写R8+读R9+机器复位", "写R80+读R80+报警清除", "写R76+读R76+主料盘修改", "写R34+读R44+XYZ1到指定点", "写R36+读R46+XYZ2到指定点", "写R3C+读R4C+XYZ1到1号编带位", "写R3E+读R4E+XYZ2到2号编带位", "写R68+读R69+XY到校正位", "写R35+读R45+Z1下降取料", "写R37+读R47+Z2下降取料", "写R3D+读R4D+Z1下降编带", "写R3F+读R4F+Z2下降编带", "写R6A+读R6B+Z轴校正位放料", "写R60+读R61+XYZ1到飞达位", "写R64+读R65+XYZ2到2号飞达位", "写R6C+读R6D+Z轴校正位取料", "写R1C+读R5C+R1轴旋转定位", "写R1F+读R5F+R2轴旋转定位", "写R62+读R63+Z1下降取料", "写R66+读R67+Z2下降取料", "写R2C+读Y1B+1号吸嘴真空", "写R2E+读Y1C+2号吸嘴真空": Mouse Down; "写R0+读R1+手动启动", "写R4+读R4+手动停止", "写R8+读R9+机器复位", "写R80+读R80+报警清除", "写R76+读R76+主料盘修改", "写R34+读R44+XYZ1到指定点", "写R36+读R46+XYZ2到指定点", "写R3C+读R4C+XYZ1到1号编带位", "写R3E+读R4E+XYZ2到2号编带位", "写R68+读R69+XY到校正位", "写R35+读R45+Z1下降取料", "写R37+读R47+Z2下降取料", "写R3D+读R4D+Z1下降编带", "写R3F+读R4F+Z2下降编带", "写R6A+读R6B+Z轴校正位放料", "写R60+读R61+XYZ1到飞达位", "写R64+读R65+XYZ2到2号飞达位", "写R6C+读R6D+Z轴校正位取料", "写R1C+读R5C+R1轴旋转定位", "写R1F+读R5F+R2轴旋转定位", "写R62+读R63+Z1下降取料", "写R66+读R67+Z2下降取料", "写R2C+读Y1B+1号吸嘴真空", "写R2E+读Y1C+2号吸嘴真空": Mouse Up {
        n166 = event-data() -> ("Type"=w417:T5, "CtlRef"=w422:refnum<vi>)  [unwired: 1 in, 6 out]
        n167 = property class="Bool"(reference=w422) -> (reference out=w418:refnum<vi>, "Label.Text"=w421:string)  [unwired: 1 in, 1 out]
        n168 = Match Pattern(string=w421, regular expression="+" ("正则表达式")) -> (before substring=w416:string)  [unwired: 1 in, 3 out]
        n169 = call "布尔复位型入队.vi"("队列输入"=w419, "数值"=w417, "控件引用"=w418, "字符消息入队列"=w416) -> ()  [unwired: 2 in, 3 out]
      }
      event "写R81+读R81+切换+快速", "写R168+读R168+切换+快速": Mouse Down {
        n170 = event-data() -> ("CtlRef"=w428:refnum<vi>)  [unwired: 1 in, 7 out]
        n171 = property class="Bool"(reference=w428) -> (reference out=w423:refnum<vi>, "Label.Text"=w427:string)  [unwired: 1 in, 1 out]
        n172 = Match Pattern(string=w427, regular expression="+" ("正则表达式")) -> (before substring=w425:string)  [unwired: 1 in, 3 out]
        n173 = call "布尔切换型入队.vi"("字符串"=w425, "true启用入队"=TRUE, "控件引用"=w423, "消息入队列"=w429) -> ()  [unwired: 8 in]
      }
      event "DT63+枚举": Value Change {
        n174 = event-data() -> ("NewVal"=w431:enum16{"90度", "180度", "270度"})  [unwired: 1 in, 5 out]
        n175 = call "字符串入队列操作.vi"("字符消息入队列"="写DT63", "数值"=w431, "界面切换队列"=w432) -> ()  [unwired: 8 in, 1 out]
      }
      event "产品界面": Mouse Down {
        n176 = event-data() -> ("CtlRef"=w435:refnum<vi>)  [unwired: 1 in, 7 out]
        n177 = call "界面切换.vi"("界面切换队列输入"=w436, "切换界面名称输入"="产品界面", "Bool引用句柄"=w435, "状态转移输入"=w437) -> ("布尔"=w433:bool)  [unwired: 7 in]
      }
      event "手动界面": Mouse Down {
        n178 = event-data() -> ("CtlRef"=w440:refnum<vi>)  [unwired: 1 in, 7 out]
        n179 = call "界面切换.vi"("界面切换队列输入"=w441, "切换界面名称输入"="手动界面", "Bool引用句柄"=w440, "状态转移输入"=w442) -> ("布尔"=w438:bool)  [unwired: 7 in]
      }
      event "手动2界面": Mouse Down {
        n180 = event-data() -> ("CtlRef"=w445:refnum<vi>)  [unwired: 1 in, 7 out]
        n181 = call "界面切换.vi"("界面切换队列输入"=w446, "切换界面名称输入"="手动2界面", "Bool引用句柄"=w445, "状态转移输入"=w447) -> ("布尔"=w443:bool)  [unwired: 7 in]
      }
      event "手动4界面": Mouse Down {
        n182 = event-data() -> ("CtlRef"=w450:refnum<vi>)  [unwired: 1 in, 7 out]
        n183 = call "界面切换.vi"("界面切换队列输入"=w451, "切换界面名称输入"="手动4界面", "Bool引用句柄"=w450, "状态转移输入"=w452) -> ("布尔"=w448:bool)  [unwired: 7 in]
      }
      event "自动界面": Mouse Down {
        n184 = event-data() -> ("CtlRef"=w455:refnum<vi>)  [unwired: 1 in, 7 out]
        n185 = call "界面切换.vi"("界面切换队列输入"=w456, "切换界面名称输入"="自动界面", "Bool引用句柄"=w455, "状态转移输入"=w457) -> ("布尔"=w453:bool)  [unwired: 7 in]
      }
      event Timeout {
        n186 = event-data() -> ()  [unwired: 1 in, 3 out]
      }
      event Panel Close? {
        n187 = event-data() -> ()  [unwired: 1 in, 4 out]
        n188 = Two Button Dialog(message="确定退出程序？" ("消息")) -> (T button?=w461:bool)  [unwired: 2 in]
        n189 = case shown="真" w461 {
          tunnel: [_ TRUE] -> w460
          tunnel: w459 -> [_ w466]
          tunnel: w458 -> [_ w465]
          frame False {
          }
          frame True {
            n190 = call "字符串入队列操作.vi"("字符消息入队列"="退出", "界面切换队列"=w465) -> ()  [unwired: 9 in, 1 out]
            n191 = call "字符串入队列操作.vi"("字符消息入队列"="写退出", "界面切换队列"=w466) -> ()  [unwired: 9 in, 1 out]
          }
        }
        n192 = event-data("Discard?"=TRUE ("放弃？")) -> ()  [unwired: 1 in, 1 out]
      }
    }
  }
  n193 = disable-structure shown="禁用" {
    frame Disabled {
      (unwired) u32 1 ("转换比例")
      (unwired) FALSE ("忽略数值上下限")
      n194 = call "布尔切换型入队.vi"() -> ()  [unwired: 12 in]
      n195 = call "批量读D+10个+16位.vi"() -> ()  [unwired: 8 in, 4 out]
      n196 = call "批量读D+5个+32位.vi"() -> ()  [unwired: 8 in, 4 out]
      n197 = call "界面切换.vi"() -> ()  [unwired: 11 in, 1 out]
      n198 = call "读D16位.vi"() -> ()  [unwired: 8 in, 4 out]
      n199 = call "写D+32位.vi"() -> ()  [unwired: 8 in, 4 out]
      n200 = call "读D32位.vi"() -> ()  [unwired: 9 in, 3 out]
      n201 = call "读触点-8位.vi"() -> ()  [unwired: 8 in, 4 out]
      n202 = call "写触点.vi"() -> ()  [unwired: 9 in, 3 out]
      n203 = call "布尔复位型入队.vi"() -> ()  [unwired: 6 in, 3 out]
      n204 = call "数值输入窗口.vi"("输入下限"=0.0, "输入上限"=9999.0, "数据类型"=enum16{"32位", "16位"}."32位") -> ("转换比例"=w472:u32)  [unwired: 9 in, 3 out]
      n205 = call "数值输入窗口.vi"() -> ()  [unwired: 13 in, 3 out]
      n206 = call "数值输入窗口.vi"() -> ()  [unwired: 13 in, 3 out]
      n207 = call "数值输入窗口.vi"() -> ()  [unwired: 13 in, 3 out]
      n208 = call "数值输入窗口.vi"() -> ()  [unwired: 13 in, 3 out]
    }
    frame Enabled {
    }
  }
  n209 = disable-structure shown="禁用" {
    frame Disabled {
      n210 = call "写D+32位.vi"() -> ()  [unwired: 8 in, 4 out]
      n211 = call "批量读D+10个+16位.vi"() -> ()  [unwired: 8 in, 4 out]
      n212 = call "写D+16位.vi"() -> ()  [unwired: 7 in, 5 out]
      n213 = call "批量读D+5个+32位.vi"() -> ()  [unwired: 8 in, 4 out]
      n214 = call "字符串入队列操作.vi"() -> ()  [unwired: 11 in, 1 out]
      n215 = call "读触点-8位.vi"() -> ()  [unwired: 8 in, 4 out]
      n216 = call "读D16位.vi"() -> ()  [unwired: 8 in, 4 out]
      n217 = call "读D32位.vi"() -> ()  [unwired: 9 in, 3 out]
      n218 = call "写触点.vi"() -> ()  [unwired: 9 in, 3 out]
      n219 = call "写触点.vi"() -> ()  [unwired: 9 in, 3 out]
    }
    frame Enabled {
    }
  }
  n220 = disable-structure shown="禁用" {
    frame Disabled {
      n221 = for {
        i -> [w474]
        n222 = case shown="9" w474 {
          frame 0, Default {
          }
          frame 1 {
          }
          frame 2 {
          }
          frame 3 {
          }
          frame 4 {
          }
          frame 5 {
          }
          frame 6 {
          }
          frame 7 {
          }
          frame 8 {
          }
          frame 9 {
          }
        }
      }
      n223 = for {
        i -> [w473]
        n224 = case shown="0, 默认" w473 {
          frame 0, Default {
          }
          frame 1 {
          }
          frame 2 {
          }
          frame 3 {
          }
          frame 4 {
          }
          frame 5 {
          }
          frame 6 {
          }
          frame 7 {
          }
        }
      }
    }
    frame Enabled {
    }
  }
  n225 = while {
    tunnel: w12 -> [w478]
    tunnel: w11 -> [w477]
    tunnel: w5 -> [w476]
    stop <- TRUE stop-if-true
    n226 = control-ref of="本VI"() -> (w475:refnum<vi>)
    n227 = Release Queue(queue=w476) -> ()  [unwired: 2 in, 3 out]
    n228 = invoke class="VI" method="FP.Close"(reference=w475) -> ()  [unwired: 2 in, 3 out]
    "VISA资源名称输出" <- w478
    "错误输出" <- w477
  }
